vi "UseMask.vi"(0 "Mask Path":path, 2 "Buffer Name Mask B/W":string, 3 "Buffer Name Mask Binary":string, 5 "Error IN":errorcluster, 8 "Width":i32, 10 "Height":i32) -> (15 "Array Mask OUT":u8[](array[numeric]), 17 "BufferMask OUT":T1, 19 "Error OUT":errorcluster)   [LabVIEW 2018]
doc: "It reads the mask in B/W format, transforms it into binary and returns the 1D array U8 of the mask and a buffer that stores memory for the mask image. It receives the path of the mask and two Strings for the desired name of the B/W mask buffer and the binary mask buffer. If you do not pass the mask route creates one, but we must pass it width and height."
uses:
  <vilib>/vision/Image Controls.llb/IMAQ Image.ctl
  <vilib>/vision/NI_Vision_Development_Module.lvlib
panel:
  out "Mask":T1(plugin-control)
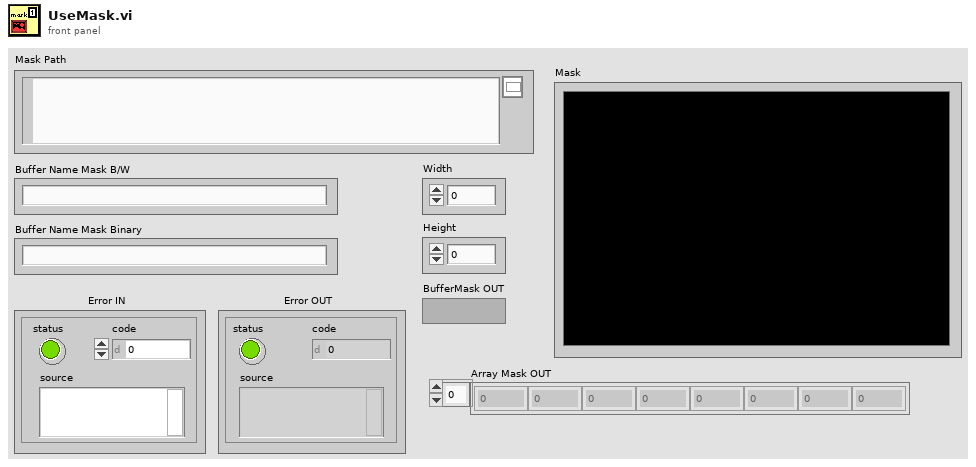
[diagram p1: front panel]
types:
  T1 = typedef "IMAQ Image.ctl" = refnum<image>
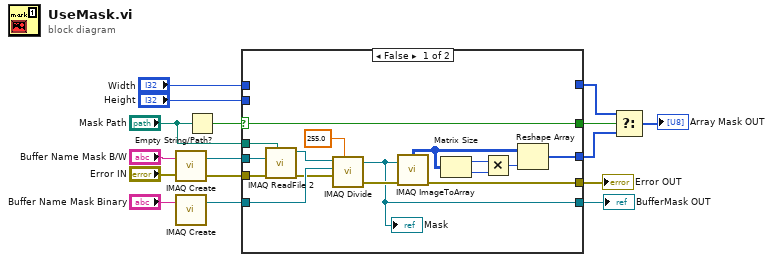
[diagram p0: block diagram]
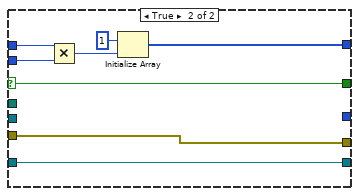
[diagram p2: hidden frame]
diagram:
  n1 = call "IMAQ Create"("Image Name"="Buffer Name Mask B/W", "error in (no error)"="Error IN") -> ("New Image"=w15:T1, "error out"=w11:errorcluster)  [unwired: 3 in]
  n2 = call "IMAQ Create"("Image Name"="Buffer Name Mask Binary") -> ("New Image"=w16:T1)  [unwired: 4 in, 1 out]
  n3 = Empty String/Path?(string/path="Mask Path") -> (empty?=w9:bool)
  n4 = case shown="False" w9 {
    selector: w9 -> [w17 w33]
    tunnel: w16 -> [w31 w39]
    tunnel: w15 -> [w30 _]
    tunnel: [w25 _] -> w13
    tunnel: w11 -> [w23 w40]
    tunnel: [w20 w40] -> w8
    tunnel: "Mask Path" -> [w19 _]
    tunnel: "Width" -> [_ w36]
    tunnel: "Height" -> [_ w35]
    tunnel: [w18 w39] -> w4
    tunnel: [_ w34] -> w3
    tunnel: [w17 w33] -> w2
    frame False {
      n5 = call "IMAQ ReadFile 2"("File Path"=w19, "error in (no error)"=w23, "Image"=w30) -> ("error out"=w22:errorcluster, "Image Out"=w29:T1)  [unwired: 4 in, 3 out]
      n6 = call "IMAQ Divide"("Image Src A"=w29, "Constant"=255.0, "Image Dst"=w31, "error in (no error)"=w22) -> ("Image Dst Out"=w18:T1, "error out"=w21:errorcluster)  [unwired: 3 in]
      "Mask" <- w18
      n7 = call "IMAQ ImageToArray"("error in (no error)"=w21, "Image"=w18) -> ("error out"=w20:errorcluster, "Image Pixels (U8)"=w26:u8[][])  [unwired: 2 in, 3 out]
      n8 = Matrix Size(0:w26) -> (1:w28:i32, 2:w27:i32)
      n9 = Multiply(x=w28, y=w27) -> (x*y=w24:i32)
      n10 = Reshape Array(w26, w24) -> (w25:u8[])
    }
    frame True {
      n11 = Multiply(x=w36, y=w35) -> (x*y=w37:i32)
      n12 = Initialize Array(u8 1 ("element"), w37) -> (w34:u8[])
    }
  }
  "Error OUT" <- w8
  "BufferMask OUT" <- w4
  n13 = Select(t=w3, s=w2, f=w13) -> (s? t:f=→"Array Mask OUT":u8[])
